vi "ReplaceDeprecatedNodes.vi"() -> ()   [LabVIEW 2024]
panel:
  out "Updated Files":path[](array[path])
  out "error out":errorcluster
  in  "Source Root Directory":path
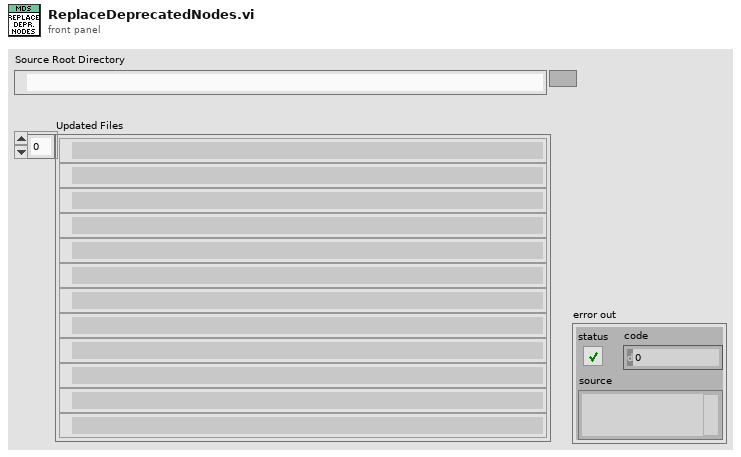
[diagram p1: front panel]
types:
  T1 = typedef "DeprecationInfo.ctl" = cluster{"NamePairs":cluster{"OldName":string, "NewName":string}[]}
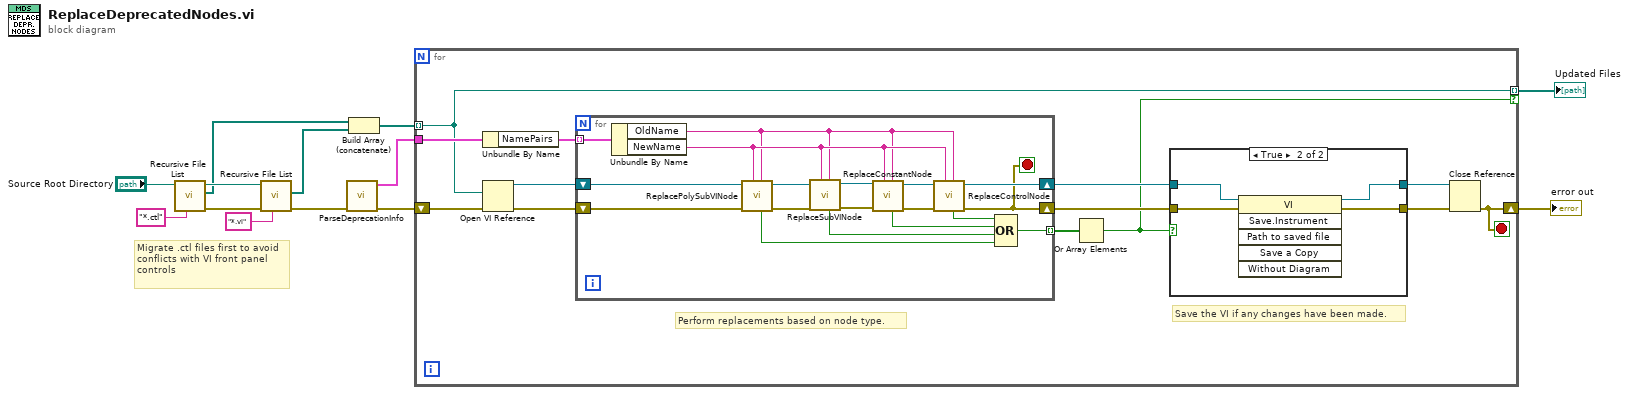
[diagram p0: block diagram]
diagram:
  # "Migrate .ctl files first to avoid conflicts with VI front panel controls"
  n1 = call <vilib>:"Recursive File List.vi"("pattern"="*.ctl", "Folder Path"="Source Root Directory") -> ("error out"=w6:errorcluster, "All Files in Dir"=w3:path[], "dup Folder Path"=w5:path)  [unwired: 5 in, 2 out]
  n2 = call <vilib>:"Recursive File List.vi"("pattern"="*.vi", "error in (no error)"=w6, "Folder Path"=w5) -> ("error out"=w10:errorcluster, "All Files in Dir"=w2:path[])  [unwired: 4 in, 3 out]
  n3 = call "ParseDeprecationInfo.vi"("error in (no error)"=w10) -> ("error out"=w12:errorcluster, "Deprecation Info"=w13:T1)  [unwired: 9 in]
  n4 = Build Array (concatenate)(w3, w2) -> (w1:path[])
  n5 = for {
    tunnel: w13 -> [w26]
    tunnel: w1 -> [w17] mode=indexing
    shift-right: [w14] -> w9
    shift-left: w12 -> [w25]
    tunnel: [w17] -> w8 mode=indexing if=w16
    stop <- w14 stop-if-true
    # "Perform replacements based on node type."
    # "Save the VI if any changes have been made."
    n6 = Unbundle By Name(w26) -> ("NamePairs"=w15:cluster{"OldName":string, "NewName":string}[])
    n7 = Open VI Reference(vi path=w17, error in (no error)=w25) -> (vi reference=w23:refnum<vi>, error out=w24:errorcluster)  [unwired: 4 in]
    n8 = for {
      tunnel: w15 -> [w44] mode=indexing
      shift-right: [w27] -> w20
      shift-left: w24 -> [w43]
      tunnel: [w35] -> w22 mode=indexing
      shift-right: [w39] -> w21
      shift-left: w23 -> [w42]
      stop <- w27 stop-if-true
      n9 = Unbundle By Name(w44) -> ("OldName"=w29:string, "NewName"=w30:string)
      n10 = call "ReplacePolySubVINode.vi"("Old File Name"=w29, "New File Name"=w30, "error in (no error)"=w43, "VI Refnum"=w42) -> ("error out"=w34:errorcluster, "VI Refnum Out"=w32:refnum<vi>, "Replaced"=w38:bool)  [unwired: 5 in]
      n11 = call "ReplaceSubVINode.vi"("Old File Name"=w29, "New File Name"=w30, "error in (no error)"=w34, "VI Refnum In"=w32) -> ("error out"=w33:errorcluster, "VI Refnum Out"=w31:refnum<vi>, "Replaced"=w28:bool)  [unwired: 5 in]
      n12 = call "ReplaceConstantNode.vi"("Old Control Name"=w29, "New Control Name"=w30, "error in (no error)"=w33, "VI Refnum In"=w31) -> ("error out"=w41:errorcluster, "VI Refnum Out"=w40:refnum<vi>, "Replaced"=w37:bool)  [unwired: 5 in]
      n13 = call "ReplaceControlNode.vi"("Old File Name"=w29, "New File Name"=w30, "error in (no error)"=w41, "VI Refnum In"=w40) -> ("error out"=w27:errorcluster, "VI Refnum Out"=w39:refnum<vi>, "Replaced"=w36:bool)  [unwired: 5 in]
      n14 = Compound Arithmetic op=OR(w36, w37, w28, w38) -> (w35:bool)
    }
    n15 = Or Array Elements(Boolean array=w22) -> (logical OR=w16:bool)
    n16 = case shown="True" w16 {
      tunnel: w21 -> [w46 w50]
      tunnel: w20 -> [w45 w49]
      tunnel: [w45 w48] -> w19
      tunnel: [w46 w47] -> w18
      frame False {
      }
      frame True {
        n17 = invoke class="VI" method="Save.Instrument"(reference=w50, error in=w49) -> (reference out=w47:refnum<vi>, error out=w48:errorcluster)  [unwired: 4 in, 4 out]
      }
    }
    n18 = Close Reference(reference=w18, error in (no error)=w19) -> (error out=w14:errorcluster)
  }
  "error out" <- w9
  "Updated Files" <- w8
